vi "(SubVI) number_SET_rule.vi"(1 "Input_2":dbl, 2 "Input_1":dbl) -> (0 "Matching_number":dbl)   [LabVIEW 2018]
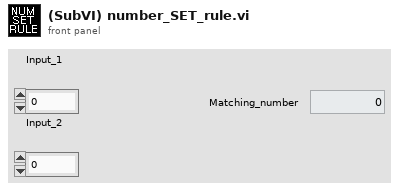
[diagram p1: front panel]
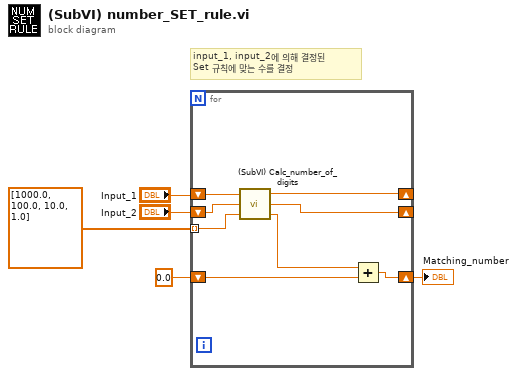
[diagram p0: block diagram]
diagram:
  # "input_1, input_2에 의해 결정된\nSet 규칙에 맞는 수를 결정"
  n1 = for {
    tunnel: dbl[] [1000.0, 100.0, 10.0, 1.0] ("digits") -> [w13] mode=indexing
    shift-right: [w10] -> _
    shift-left: "Input_1" -> [w12]
    shift-right: [w9] -> _
    shift-left: "Input_2" -> [w11]
    shift-right: [w8] -> w1
    shift-left: 0.0 -> [w6]
    n2 = call "(SubVI) Calc_number_of_digits.vi"("target_digit"=w13, "Input_2"=w11, "Input_1"=w12) -> ("output_digit"=w7:dbl, "remain_2"=w9:dbl, "remain_1"=w10:dbl)
    n3 = Add(x=w7, y=w6) -> (x+y=w8:dbl)
  }
  "Matching_number" <- w1
